vi "Motor State Toggle.vi"(0 "MotorControlDevRef":T1={"DeviceStatus"={"status"=FALSE, "code"=0, "source"=""}, "Type"=enum."PWM", "PWM"={"PWM Channel"=enum."Invalid", "DeadBand"={"Name"="", "maxPositivePwm"=0, "minPositivePwm"=0, "centerPwm"=0, "maxNegativePwm"=0, "minNegativePwm"=0, "angularRange"=0}}, "CAN"={"Device Number"=0, "Control Mode"=enum."Percent VBus", "Semaphore"=refnum, "Max Vout"=12.0, "TalonSRX Control Mode"=enum."Percent VBus"}, "Invert"=FALSE}, 1 "EncoderDevRef":T8={"DevStatus"={"status"=FALSE, "code"=0, "source"=""}, "EncoderIndex"=enum."Invalid", "CounterIndex"=enum."Ctr 1", "DistancePerCount"=2.0, "Decoding Type"=enum."4x"}, 2 "Upper Limit":dbl, 3 "Motor Speed":dbl, 4 "Switch States":bool, 5 "Lower Limit":dbl) -> (15 "At Upper Limit":bool, 16 "Distance":dbl, 18 "At Lower Limit":bool)   [LabVIEW 2015]
uses:
  <vilib>/Rock Robotics/WPI/Encoder/WPI_EncoderDevRef.ctl
  <vilib>/Rock Robotics/SystemInterfaces/Encoder/FPGA_EncoderIdx.ctl
  <vilib>/Rock Robotics/SystemInterfaces/Counter/FPGA_CounterCtrSystemIndex.ctl
  <vilib>/Rock Robotics/WPI/Encoder/WPI_EncoderType.ctl
  <vilib>/Rock Robotics/WPI/MotorControl/WPI_MotorControlDeviceRef.ctl
  <vilib>/Rock Robotics/WPI/MotorControl/WPI_MotorControlType.ctl
  <vilib>/Rock Robotics/SystemInterfaces/DIO/FPGA_DIOPWMChannel.ctl
  <vilib>/Rock Robotics/WPI/PWM/WPI_PWMDeadband.ctl
  <vilib>/Rock Robotics/WPI/CAN/Jaguar/SubVIs/WPI_CANJaguar_ControlMode.ctl
  <vilib>/Rock Robotics/WPI/CAN/TalonSRX/WPI_CANTalonSRX_APIControlMode.ctl
panel:
  out "Motor Output":dbl
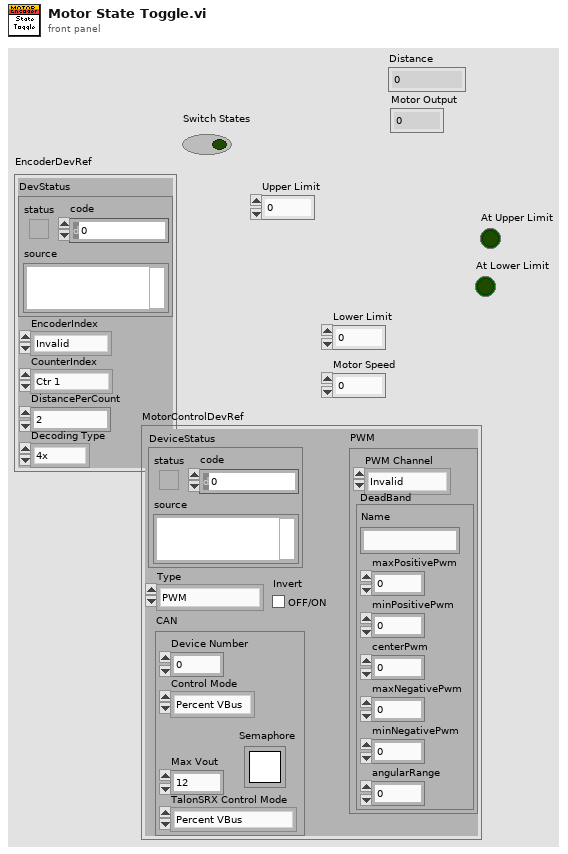
[diagram p1: front panel]
types:
  T1 = typedef "WPI_MotorControlDeviceRef.ctl" = cluster{"DeviceStatus":errorcluster, "Type":T2, "PWM":cluster{"PWM Channel":T3, "DeadBand":T4}, "CAN":cluster{"Device Number":u8, "Control Mode":T5, "Semaphore":T6, "Max Vout":dbl, "TalonSRX Control Mode":T7}, "Invert":bool}
  T2 = typedef "WPI_MotorControlType.ctl" = enum16{"PWM", "CAN", "CANTalonSRX"}
  T3 = typedef "FPGA_DIOPWMChannel.ctl" = enum8{"PWM 0", "PWM 1", "PWM 2", "PWM 3", "PWM 4", "PWM 5", "PWM 6", "PWM 7", "PWM 8", "PWM 9", "PWM MXP 0", "PWM MXP 1", "PWM MXP 2", "PWM MXP 3", "PWM MXP 4", "PWM MXP 5", "PWM MXP 6", "PWM MXP 7", "PWM MXP 8", "PWM MXP 9", "Invalid"}
  T4 = typedef "WPI_PWMDeadband.ctl" = cluster{"Name":string, "maxPositivePwm":i32, "minPositivePwm":i32, "centerPwm":i32, "maxNegativePwm":i32, "minNegativePwm":i32, "angularRange":u16}
  T5 = typedef "WPI_CANJaguar_ControlMode.ctl" = enum8{"Percent VBus", "Current", "Speed", "Position", "Voltage"}
  T6 = typedef "Semaphore RefNum" = refnum<k1>
  T7 = typedef "WPI_CANTalonSRX_APIControlMode.ctl" = enum8{"Percent VBus", "Speed", "Position", "Slave", "Unchanged / Invalid", "Voltage Compensation", "Current", "Motion Profile"}
  T8 = typedef "WPI_EncoderDevRef.ctl" = cluster{"DevStatus":errorcluster, "EncoderIndex":T9, "CounterIndex":T10, "DistancePerCount":dbl, "Decoding Type":T11}
  T9 = typedef "FPGA_EncoderIdx.ctl" = enum8{"Enc 0", "Enc 1", "Enc 2", "Enc 3", "Enc 4", "Enc 5", "Enc 6", "Enc 7", "Invalid"}
  T10 = typedef "FPGA_CounterCtrSystemIndex.ctl" = enum8{"Ctr 0", "Ctr 1", "Ctr 2", "Ctr 3", "Ctr 4", "Ctr 5", "Ctr 6", "Ctr 7", "Invalid"}
  T11 = typedef "WPI_EncoderType.ctl" = enum16{"1x", "2x", "4x"}
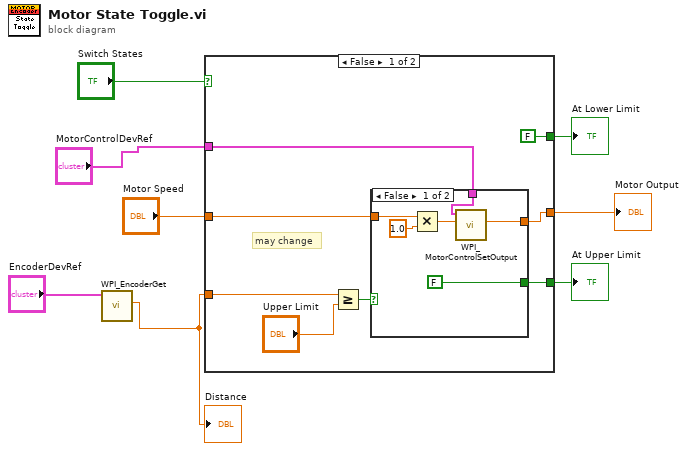
[diagram p0: block diagram]
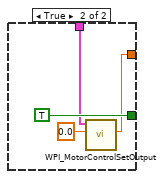
[diagram p2: hidden frame]
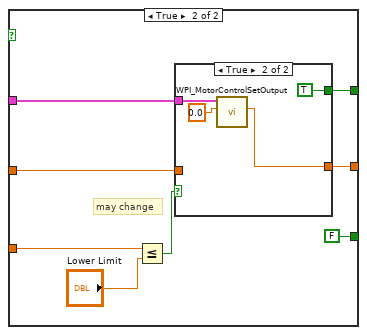
[diagram p3: hidden frame]
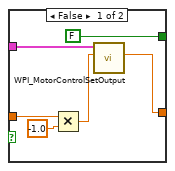
[diagram p4: hidden frame]
diagram:
  n1 = call <vilib>:"WPI_EncoderGet.vi"("EncoderDevRef"="EncoderDevRef") -> ("Distance"=w4:dbl)  [unwired: 5 in, 5 out]
  "Distance" <- w4
  n2 = case shown="False" "Switch States" {
    tunnel: w4 -> [w14 w33]
    tunnel: "Motor Speed" -> [w13 w31]
    tunnel: "MotorControlDevRef" -> [w10 w30]
    tunnel: [w12 FALSE] -> w7
    tunnel: [FALSE ("At Lower Limit") w28] -> w6
    tunnel: [w9 w27] -> w2
    frame False {
      # "may change"
      n3 = Greater Or Equal?(x=w14, y="Upper Limit") -> (x >= y?=w15:bool)
      n4 = case shown="False" w15 {
        tunnel: w13 -> [w20 _]
        tunnel: [FALSE TRUE] -> w12
        tunnel: w10 -> [w18 w24]
        tunnel: [w17 w23] -> w9
        frame False {
          n5 = Multiply(x=w20, y=1.0) -> (x*y=w21:dbl)
          n6 = call <vilib>:"WPI_MotorControlSetOutput.vi"("Output"=w21, "MotorControlDevRef"=w18) -> ("Motor Output"=w17:dbl)  [unwired: 7 in, 2 out]
        }
        frame True {
          n7 = call <vilib>:"WPI_MotorControlSetOutput.vi"("Output"=0.0, "MotorControlDevRef"=w24) -> ("Motor Output"=w23:dbl)  [unwired: 7 in, 2 out]
        }
      }
    }
    frame True {
      # "may change"
      n8 = Less Or Equal?(x=w33, y="Lower Limit") -> (x <= y?=w32:bool)
      n9 = case shown="True" w32 {
        tunnel: w31 -> [w38 _]
        tunnel: w30 -> [w37 w43]
        tunnel: [FALSE ("At Lower Limit") TRUE] -> w28
        tunnel: [w35 w41] -> w27
        frame False {
          n10 = Multiply(x=w38, y=-1.0) -> (x*y=w39:dbl)
          n11 = call <vilib>:"WPI_MotorControlSetOutput.vi"("Output"=w39, "MotorControlDevRef"=w37) -> ("Motor Output"=w35:dbl)  [unwired: 7 in, 2 out]
        }
        frame True {
          n12 = call <vilib>:"WPI_MotorControlSetOutput.vi"("Output"=0.0, "MotorControlDevRef"=w43) -> ("Motor Output"=w41:dbl)  [unwired: 7 in, 2 out]
        }
      }
    }
  }
  "At Lower Limit" <- w6
  "At Upper Limit" <- w7
  "Motor Output" <- w2
